vi "Write.vi"(8 "Error In":errorcluster, 10 "Write Buffer":string, 11 "VISA resource name":refnum<visa-resource-name>) -> (0 "Error Out":errorcluster, 3 "VISA resource name out":refnum<visa-resource-name>)   [LabVIEW 2013]
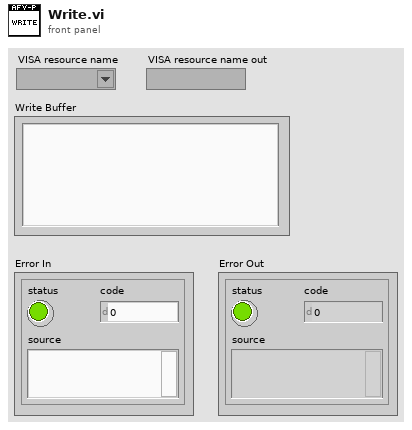
[diagram p1: front panel]
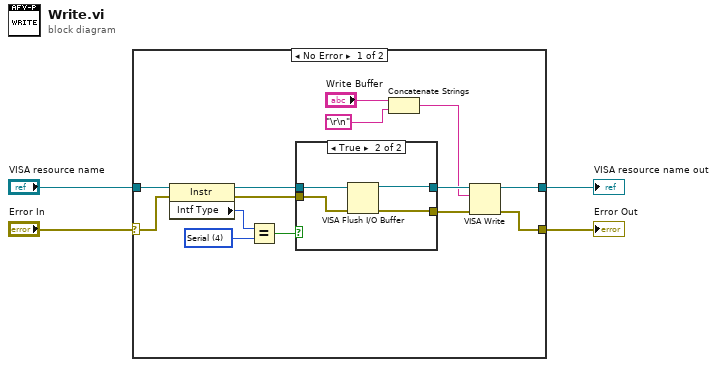
[diagram p0: block diagram]
diagram:
  n1 = case shown="No Error" "Error In" {
    selector: "Error In" -> [w11 w26]
    tunnel: [w6 w26] -> w3
    tunnel: "VISA resource name" -> [w12 w25]
    tunnel: [w5 w25] -> w1
    frame No Error {
      w13 = u16 4 items=["GPIB"=1, "VXI"=2, "GPIB-VXI"=3, "Serial"=4, "PXI"=5, "TCPIP"=6, "USB"=7, "FireWire"=9] ("Interface Information:Interface Type")
      n2 = property class="Instr"(reference=w12, error in=w11) -> (reference out=w9:refnum<visa-resource-name>, error out=w10:errorcluster, "Intf Type"=w8:u16)
      n3 = Equal?(x=w8, y=w13) -> (x = y?=w7:bool)
      n4 = case shown="True" w7 {
        tunnel: w9 -> [w20 w24]
        tunnel: [w19 w21] -> w18
        tunnel: [w20 w22] -> w17
        tunnel: w10 -> [w19 w23]
        frame False {
        }
        frame True {
          n5 = VISA Flush I/O Buffer(VISA resource name=w24, error in (no error)=w23) -> (VISA resource name out=w22:refnum<visa-resource-name>, error out=w21:errorcluster)  [unwired: 1 in]
        }
      }
      n6 = Concatenate Strings("Write Buffer", "\r\n") -> (w15:string)
      n7 = VISA Write(VISA resource name=w17, write buffer=w15, error in (no error)=w18) -> (VISA resource name out=w5:refnum<visa-resource-name>, error out=w6:errorcluster)  [unwired: 1 out]
    }
    frame Error {
    }
  }
  "Error Out" <- w3
  "VISA resource name out" <- w1
